vi "test_PipelineResult_Encode_and_decode.vi"() -> ()   [LabVIEW 2020]
uses:
  PhotonVisionLib/TypeDef/PhotonPipelineResultType.ctl
  PhotonVisionLib/TypeDef/PhotonTrackedTargetType.ctl
  PhotonVisionLib/TypeDef/TargetCornerType.ctl
  <vilib>/Rock Robotics/WPI/ThirdParty/JAS_Junk/TrajLib/TypeDef/TRANSFORM2D.ctl
  <vilib>/Rock Robotics/WPI/ThirdParty/JAS_Junk/TrajLib/TypeDef/TRANSLATION2D.ctl
  <vilib>/Rock Robotics/WPI/ThirdParty/JAS_Junk/TrajLib/TypeDef/ROTATION2D.ctl
  PhotonVisionLib/PhotonVisionLib.lvlib
  <vilib>/Rock Robotics/WPI/ThirdParty/JAS_Junk/TrajLib/Trajectory_Library.lvlib
panel:
  in  "FiducialId":i32
  in  "Pitch":dbl
  in  "Area":dbl
  in  "Skew":dbl
  in  "CameraToTarget":T1={"TRANSLATION"={"X"=0.0, "Y"=0.0}, "ROTATION"={"VALUE"=0.0, "COS"=1.0, "SIN"=0.0}, "xF"=FALSE} {"ROTATION"."SIN" format="%13.4f"; "ROTATION"."COS" format="%13.4f"; "ROTATION"."VALUE" format="%13.4f"; "TRANSLATION"."Y" format="%14.3f"; "TRANSLATION"."X" format="%14.3f"}
  in  "Yaw":dbl
  in  "TargetCorners":T4[](array[typedef])
  in  "Latency_Millis":dbl
  out "Packet_RawData":u8[](array[numeric])
  out "Pipeline In":T5 {"Targets"."CameraToTarget"."ROTATION"."SIN" format="%13.4f"; "Targets"."CameraToTarget"."ROTATION"."COS" format="%13.4f"; "Targets"."CameraToTarget"."ROTATION"."VALUE" format="%13.4f"; "Targets"."CameraToTarget"."TRANSLATION"."Y" format="%14.3f"; "Targets"."CameraToTarget"."TRANSLATION"."X" format="%14.3f"}
  out "Pipeline Out":T5 {"Targets"."CameraToTarget"."ROTATION"."SIN" format="%13.4f"; "Targets"."CameraToTarget"."ROTATION"."COS" format="%13.4f"; "Targets"."CameraToTarget"."ROTATION"."VALUE" format="%13.4f"; "Targets"."CameraToTarget"."TRANSLATION"."Y" format="%14.3f"; "Targets"."CameraToTarget"."TRANSLATION"."X" format="%14.3f"}
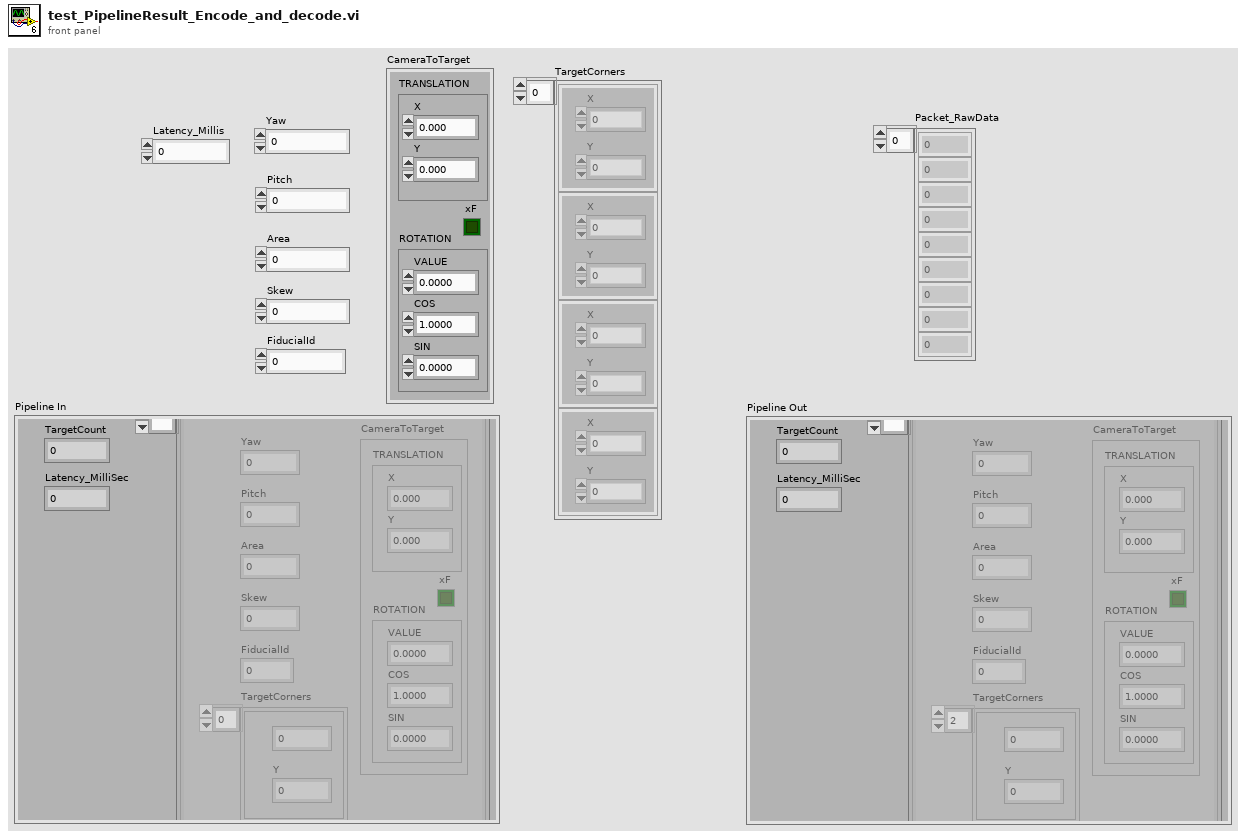
[diagram p1: front panel]
types:
  T1 = typedef "Trajectory_Library.lvlib/TRANSFORM2D.ctl" = cluster{"TRANSLATION":T2, "ROTATION":T3, "xF":bool}
  T2 = typedef "Trajectory_Library.lvlib/TRANSLATION2D.ctl" = cluster{"X":dbl, "Y":dbl}
  T3 = typedef "Trajectory_Library.lvlib/ROTATION2D.ctl" = cluster{"VALUE":dbl, "COS":dbl, "SIN":dbl}
  T4 = typedef "PhotonVisionLib.lvlib/TargetCornerType.ctl" = cluster{"X":dbl, "Y":dbl}
  T5 = typedef "PhotonVisionLib.lvlib/PhotonPipelineResultType.ctl" = cluster{"TargetCount":i32, "Latency_MilliSec":dbl, "Targets":T6[]}
  T6 = typedef "PhotonVisionLib.lvlib/PhotonTrackedTargetType.ctl" = cluster{"Yaw":dbl, "Pitch":dbl, "Area":dbl, "Skew":dbl, "TargetCorners":T4[], "CameraToTarget":T1, "FiducialId":i32}
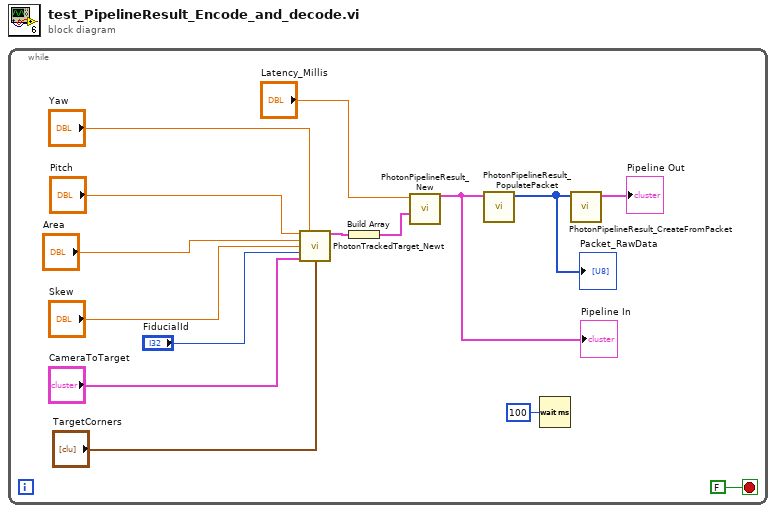
[diagram p0: block diagram]
diagram:
  n1 = while {
    stop <- FALSE stop-if-true
    n2 = call "PhotonTrackedTarget_Newt.vi"("Pitch"="Pitch", "Yaw"="Yaw", "Area"="Area", "Skew"="Skew", "FiducalId"="FiducialId", "CameraToTarget"="CameraToTarget", "TargetCorners"="TargetCorners") -> ("TrackedTarget"=w12:T6)  [unwired: 8 in]
    n3 = Build Array(w12) -> (w11:T6[])
    n4 = call "PhotonPipelineResult_New.vi"("TrackedTargets"=w11, "Latency_Millis"="Latency_Millis") -> ("PhotonPipelineResult"=w10:T5)  [unwired: 9 in]
    "Pipeline In" <- w10
    n5 = call "PhotonPipelineResult_PopulatePacket.vi"("PhotonPipelineResult"=w10) -> ("Packet_RawData"=w9:u8[])  [unwired: 10 in]
    "Packet_RawData" <- w9
    n6 = Wait (ms)(milliseconds to wait=u32 100) -> ()  [unwired: 1 out]
    n7 = call "PhotonPipelineResult_CreateFromPacket.vi"("RawData"=w9) -> ("PhotonPipelineResult"=→"Pipeline Out":T5)  [unwired: 10 in]
  }
